vi "Initialize (FPGA).vi"(8 "error in (no error)":errorcluster, 10 "Actuator ID (0)":i32, 11 "FPGA VI Reference":refnum<k20>) -> (0 "error out":errorcluster, 3 "Hitec HS400 Series out":refnum<class "Hitec HS400 Series.lvclass">)   [LabVIEW 2013, in "Hitec HS400 Series FPGA.lvclass"]
doc: "Establishes communication with the sensor. Therefore, call this VI before calling other sensor driver VIs for this sensor. Generally, you need to call the Initialize VI only once at the beginning of an application.\n\n<B>Notes:</B>\nPlease refer to the example project in the FPGA Example folder of this driver for how to configure the FPGA target and use this VI."
uses:
  Hitec HS400 Series FPGA.lvclass
  Hitec HS400 Series.lvclass
  Hitec HS400 Series FPGA.lvclass/Hitec HS400 Series FPGA.ctl
panel:
  # "(c) 2011 National Instruments.  ALL RIGHTS RESERVED."
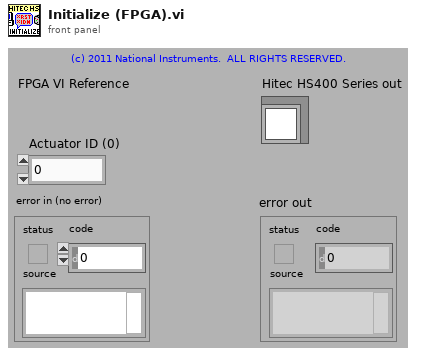
[diagram p1: front panel]
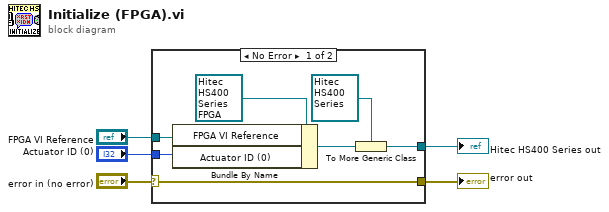
[diagram p0: block diagram]
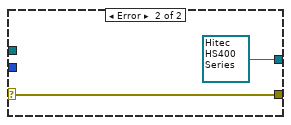
[diagram p2: hidden frame]
diagram:
  n1 = case shown="No Error" "error in (no error)" {
    selector: "error in (no error)" -> [w10 w14]
    tunnel: "FPGA VI Reference" -> [w11 _]
    tunnel: [w10 w14] -> w3
    tunnel: [w7 refnum<class "Hitec HS400 Series.lvclass"> refnum ("Parallax Standard Servo.lvclass")] -> w2
    tunnel: "Actuator ID (0)" -> [w6 _]
    frame No Error {
      n2 = Bundle By Name(cluster=refnum<class "Hitec HS400 Series FPGA.lvclass"> refnum ("Parallax Standard Servo FPGA in"), "FPGA VI Reference"=w11, "Actuator ID (0)"=w6) -> (w9:refnum<class "Hitec HS400 Series FPGA.lvclass">)
      n3 = To More Generic Class(target class=refnum<class "Hitec HS400 Series.lvclass"> refnum ("Parallax Standard Servo.lvclass"), reference=w9) -> (generic class reference=w7:refnum<class "Hitec HS400 Series.lvclass">)
    }
    frame Error {
    }
  }
  "Hitec HS400 Series out" <- w2
  "error out" <- w3
